vi "CTRE_Phoenix_CANdle_SetTwoSizeAnimation.vi"(0 "CTRE_CANdle_DeviceRef":T2, 5 "idx":i32, 7 "speed":dbl, 9 "numLED":i32, 11 "error in":errorcluster, 12 "LED Color":T1, 13 "direction":i32, 14 "size":i32) -> (4 "CTRE_CANdle_DeviceRef":T2, 15 "error out":errorcluster)   [LabVIEW 2020]
uses:
  <vilib>/Rock Robotics/WPI/ThirdParty/Phoenix-LabVIEW/CANdle/Controls/CTRE_Phoenix_CANdle_DeviceRef.ctl
  <vilib>/Rock Robotics/WPI/ThirdParty/Phoenix-LabVIEW/CANdle/Controls/CTRE_Phoenix_CANdle_LEDColor.ctl
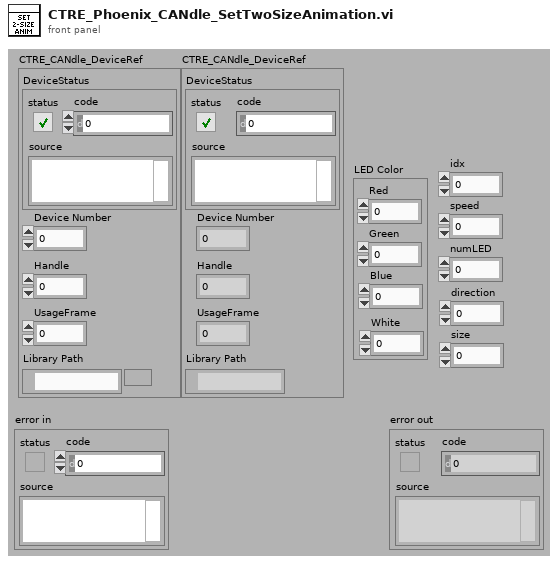
[diagram p1: front panel]
types:
  T1 = typedef "CTRE_Phoenix_CANdle_LEDColor.ctl" = cluster{"Red":u8, "Green":u8, "Blue":u8, "White":u8}
  T2 = typedef "CTRE_Phoenix_CANdle_DeviceRef.ctl" = cluster{"DeviceStatus":errorcluster, "Device Number":u8, "Handle":u64, "UsageFrame":u32, "Library Path":path}
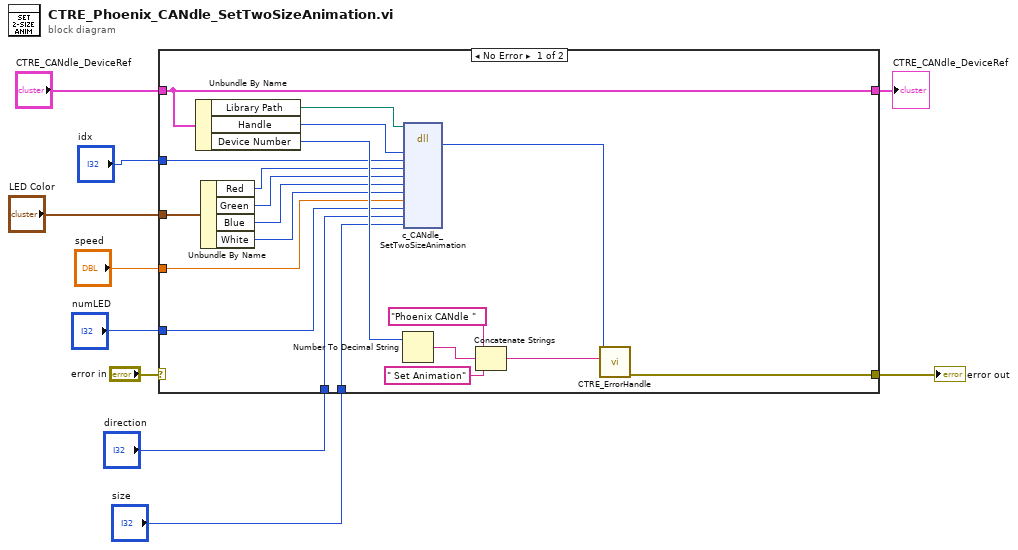
[diagram p0: block diagram]
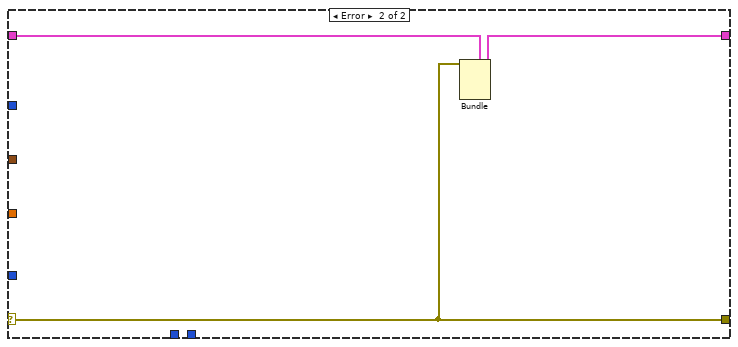
[diagram p2: hidden frame]
diagram:
  n1 = case shown="No Error" "error in" {
    selector: "error in" -> [_ w32]
    tunnel: "CTRE_CANdle_DeviceRef" -> [w24 w33]
    tunnel: [w30 w32] -> w10
    tunnel: [w24 w31] -> w7
    tunnel: "idx" -> [w20 _]
    tunnel: "speed" -> [w19 _]
    tunnel: "numLED" -> [w18 _]
    tunnel: "LED Color" -> [w17 _]
    tunnel: "direction" -> [w12 _]
    tunnel: "size" -> [w11 _]
    frame No Error {
      n2 = Unbundle By Name(w24) -> ("Library Path"=w22:path, "Handle"=w21:u64, "Device Number"=w23:u8)
      n3 = Unbundle By Name(w17) -> ("Red"=w16:u8, "Green"=w15:u8, "Blue"=w14:u8, "White"=w13:u8)
      n4 = Number To Decimal String(number=w23) -> (decimal integer string=w28:string)  [unwired: 1 in]
      n5 = dll-call lib="?" fn="c_CANdle_SetTwoSizeAnimation"(path in=w22, "handle"=w21, "idx"=w20, "r"=w16, "g"=w15, "b"=w14, "w"=w13, "speed"=w19, "numLED"=w18, "direction"=w12, "size"=w11) -> ("return type"=w26:i32)  [unwired: 12 in, 2 out]
      n6 = Concatenate Strings("Phoenix CANdle " ("string"), w28, " Set Animation" ("string")) -> (w25:string)
      n7 = call <vilib>:"CTRE_ErrorHandle.vi"("origin"=w25, "code"=w26) -> ("error out"=w30:errorcluster)  [unwired: 9 in]
    }
    frame Error {
      n8 = Bundle(cluster=w33, "DeviceStatus"=w32) -> (w31:T2)  [unwired: 4 in]
    }
  }
  "error out" <- w10
  "CTRE_CANdle_DeviceRef" <- w7
